vi "CSConnectGUI.update listbox.vi"(0 "listbox":refnum<vi>, 1 "channelNames":string[](array[string]), 2 "nomVoltage":dbl[](array[numeric]), 3 "actOutVoltages":dbl[][](array[numeric]), 4 "nomOutVoltages":dbl[][](array[numeric]), 5 "error in (no error)":errorcluster, 7 "NumberOutChannels":i32, 9 "DIMInterface <> Variable":T1(array[cluster]), 11 "actStatus":i32[][](array[numeric]), 13 "ConnectionMatrix":bool[][](array[boolean])) -> (19 "error out":errorcluster)   [LabVIEW 2014, in "CSConnectGUI.lvlib"]
doc: "Displays data of the PowerSupply in advanced mode."
uses:
  CSConnectGUI.lvlib
  CSlibraries/UtilityLib/UtilityLib.lvlib
  CS_Core/CSApplicationBaseClasses/PSChannelBase/PSChannelBase.lvlib
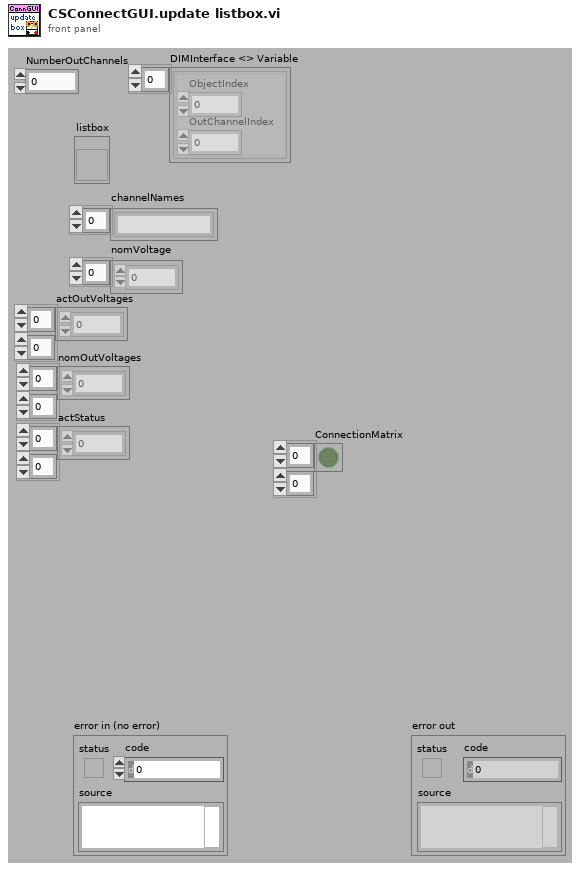
[diagram p1: front panel]
types:
  T1 = cluster{"ObjectIndex":i32, "OutChannelIndex":i32}[]
  T2 = typedef "UtilityLib.lvlib/UtilityLib.valueStatus.ctl" = enum16{"no info available", "stand by/off", "on", "warning", "alarm/malfunction", "not implemented", "user action required", "important information", "system default", "control default", "indicator default", "button default"}
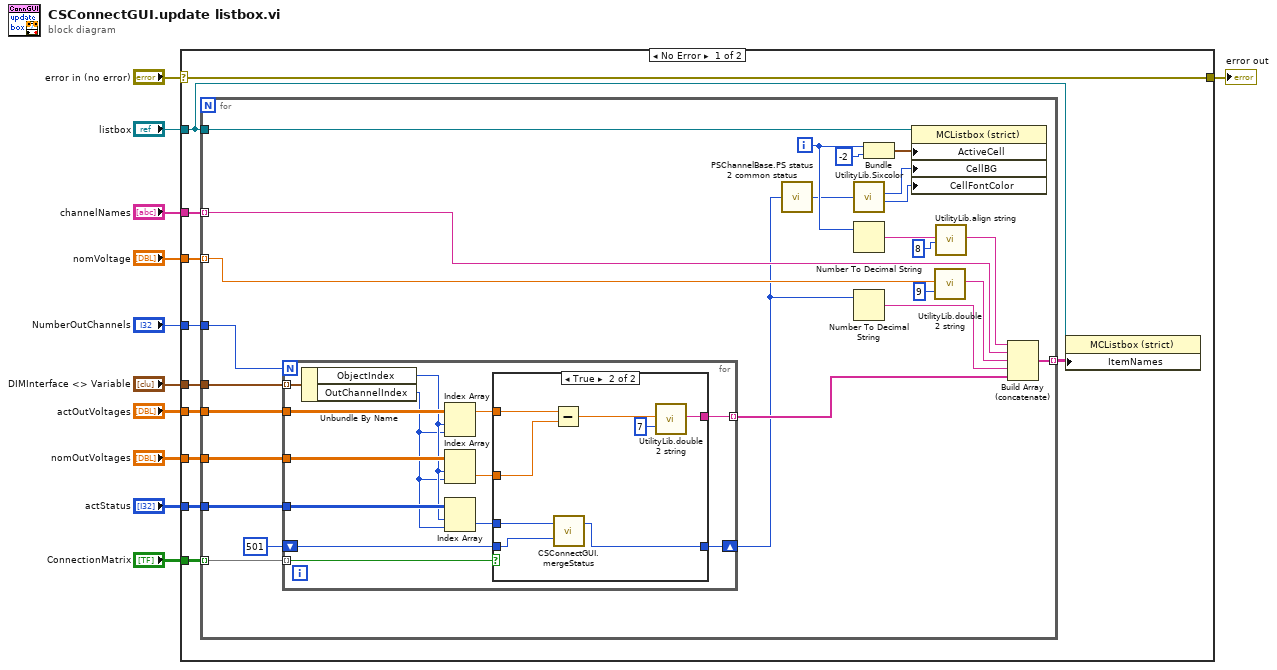
[diagram p0: block diagram]
diagram:
  n1 = case shown="No Error" "error in (no error)" {
    selector: "error in (no error)" -> [w19 w70]
    tunnel: [w19 w70] -> w10
    tunnel: "channelNames" -> [w22 _]
    tunnel: "nomVoltage" -> [w21 _]
    tunnel: "listbox" -> [w18 _]
    tunnel: "NumberOutChannels" -> [w17 _]
    tunnel: "actOutVoltages" -> [w16 _]
    tunnel: "ConnectionMatrix" -> [w15 _]
    tunnel: "DIMInterface <> Variable" -> [w14 _]
    tunnel: "nomOutVoltages" -> [w13 _]
    tunnel: "actStatus" -> [w12 _]
    frame No Error {
      n2 = for {
        tunnel: w22 -> [w47] mode=indexing
        tunnel: w21 -> [w46] mode=indexing
        tunnel: [w44] -> w20 mode=indexing
        tunnel: w18 -> [w43]
        tunnel: w17 -> [w32]
        tunnel: w16 -> [w29]
        tunnel: w15 -> [w28] mode=indexing
        tunnel: w14 -> [w27]
        tunnel: w13 -> [w26]
        tunnel: w12 -> [w25]
        i -> [w40]
        n3 = for {
          N: w32 -> [_]
          tunnel: [w60] -> w31 mode=indexing
          tunnel: w29 -> [w59]
          tunnel: w28 -> [w58] mode=indexing
          tunnel: w27 -> [w56] mode=indexing
          tunnel: w26 -> [w55]
          tunnel: w25 -> [w53]
          shift-right: [w48] -> w23
          shift-left: 501 ("number") -> [w49]
          n4 = Unbundle By Name(w56) -> ("ObjectIndex"=w52:i32, "OutChannelIndex"=w51:i32)
          n5 = Index Array(array=w59, index (row)=w52, index (col)=w51) -> (element=w57:dbl)
          n6 = Index Array(array=w55, index (row)=w52, index (col)=w51) -> (element=w54:dbl)
          n7 = Index Array(array=w53, index (row)=w52, index (col)=w51) -> (element=w50:i32)
          n8 = case shown="True" w58 {
            tunnel: [_ w68] -> w60
            tunnel: w57 -> [_ w67]
            tunnel: w54 -> [_ w65]
            tunnel: w50 -> [_ w64]
            tunnel: w49 -> [w61 w63]
            tunnel: [w61 w62] -> w48
            frame False {
            }
            frame True {
              n9 = Subtract(x=w67, y=w65) -> (x-y=w66:dbl)
              n10 = call "CSConnectGUI.mergeStatus.vi"("Input1"=w64, "Input2"=w63) -> ("Out"=w62:i32)  [unwired: 17 in]
              n11 = call "UtilityLib.double 2 string.vi"("Numeric"=w66, "length"=u8 7) -> ("String"=w68:string)  [unwired: 16 in, 1 out]
            }
          }
        }
        n12 = call "PSChannelBase.PS status 2 common status .vi"("PSStatus"=w23) -> ("commonStatus"=w34:T2)  [unwired: 4 in]
        n13 = call "UtilityLib.Sixcolor.vi"("State"=w34) -> ("elementBackground"=w39:u32, "elementText"=w35:u32)  [unwired: 2 in, 2 out]
        n14 = Number To Decimal String(number=w40) -> (decimal integer string=w38:string)  [unwired: 1 in]
        n15 = Number To Decimal String(number=w23) -> (decimal integer string=w33:string)  [unwired: 1 in]
        n16 = Bundle(w40, -2) -> (w42:cluster{i32, i32})  [unwired: 1 in]
        n17 = property class="MCListbox (strict)"(reference=w43, "ActiveCell"=w42, "CellBG"=w39, "CellFontColor"=w35) -> ()  [unwired: 1 in, 2 out]
        n18 = call "UtilityLib.double 2 string.vi"("Numeric"=w46, "length"=u8 9) -> ("String"=w45:string)  [unwired: 16 in, 1 out]
        n19 = call "UtilityLib.align string.vi"("stringIn"=w38, "stringLength (80)"=u16 8) -> ("stringOut"=w37:string)  [unwired: 16 in, 1 out]
        n20 = Build Array (concatenate)(w37, w47, w45, w33, w31) -> (w44:string[])
      }
      n21 = property class="MCListbox (strict)"(reference=w18, "ItemNames"=w20) -> ()  [unwired: 1 in, 2 out]
    }
    frame Error {
    }
  }
  "error out" <- w10
